vi "Set Numeric Control Value (Array).vi"(9 "New values":dbl[](array[numeric]), 11 "Digital Contol refs":refnum<vi>[](array[refnum])) -> (0 "error out":errorcluster, 3 "Digital Control refs out":refnum<vi>[](array[refnum]))   [LabVIEW 2021, in "Settings.lvlib"]
doc: "Set new values on the digital controls according to the sequence in the arrays."
uses:
  Settings.lvlib
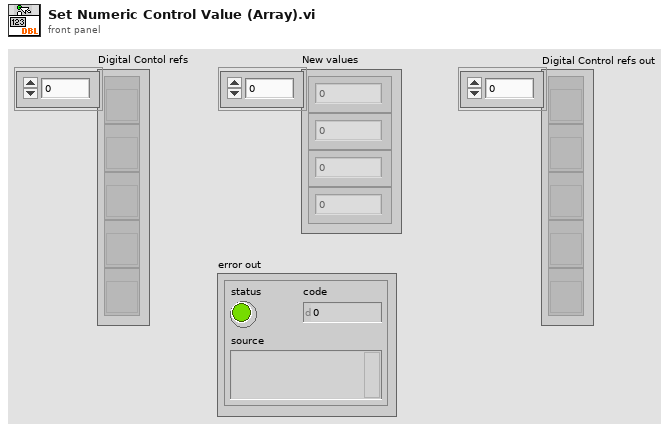
[diagram p1: front panel]
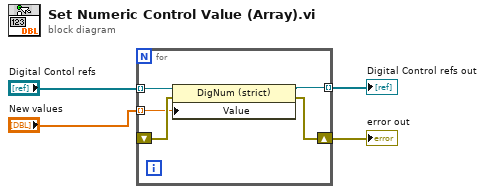
[diagram p0: block diagram]
diagram:
  n1 = for {
    tunnel: "Digital Contol refs" -> [w9] mode=indexing
    tunnel: "New values" -> [w5] mode=indexing
    shift-right: [w8] -> w2
    shift-left: _ -> [w7]
    tunnel: [w6] -> w1 mode=indexing
    n2 = property class="DigNum (strict)"(reference=w9, error in=w7, "Value"=w5) -> (reference out=w6:refnum<vi>, error out=w8:errorcluster)
  }
  "error out" <- w2
  "Digital Control refs out" <- w1
